vi "ADC SNR_new - Copy.vi"(8 "error in (no error)":errorcluster, 9 "Sequence parameters":string[][](array[string])=[["Min limit", "Max limit", "Register sheet file", "Register Sheet"], ["", "", "CC2600.xls", "TX_BLE;Trim"], ["Reg write (addr;value)", "Operating frequency [Hz]", "", ""], ["NA", "2.44G", "", ""]], 10 "Run type":i32, 11 "Method parameters":T4={"Dev"={"Do not disturb DUT"=FALSE, "XOSC"=32000000.0, "Board type"="", "EM"="", "Configure tempboard"=TRUE, "Device specific info"=[], "Generic Object"=refnum}, "Method"={"Run type"=1, "Test name"="Current LPM2 4", "Comment"="", "Results folder"="", "AFC"=enum."Off", "Method name"="Current LPM2 4", "Method results"={"Excel brief report"=FALSE, "Spotfire report"=FALSE, "Starfish report"=FALSE}, "Operator"="", "Reference time"=timestamp(0 s since 1904-01-01), "AFC delay"=0.0, "Initialization"=enum."Enabled", "MD5 Sum"="", "HW addon board"=enum."None", "AFC Regsheet"="", "AFC Regfile"=path "", "dummy"=0.0}, "Inst"={"Instr"={"PS1"={"Name"="", "GPIB address"="", "VISA session"=""}, "PS2"={"Name"="", "GPIB address"="", "VISA session"=""}, "TC1"={"Name"="", "GPIB address"="", "VISA session"=""}, "TC2"={"Name"="", "GPIB address"="", "VISA session"=""}, "SA1"={"Name"="", "GPIB address"="", "VISA session"=""}, "SA2"={"Name"="", "GPIB address"="", "VISA session"=""}, "SG1"={"Name"="", "GPIB address"="", "VISA session"=""}, "SG2"={"Name"="", "GPIB address"="", "VISA session"=""}, "SG3"={"Name"="", "GPIB address"="", "VISA session"=""}, "MI1"={"Name"="", "GPIB address"="", "VISA session"=""}, "MI2"={"Name"="", "GPIB address"="", "VISA session"=""}, "SW SA"={"Name"="", "Controller addr"=""}, "SW SG"={"Name"="", "Controller addr"=""}, "MI3"={"Name"="", "GPIB address"="", "VISA session"=""}}, "Switchbox"={"RF Path"=0, "Cal compensation"=enum."TX", "Switchbox gain mode"="", "State"=enum."TX"}, "Instr to control (i.e. SA1)"="Default", "Intrument info string"=""}, "Sequence parameters"=[["Weight", "Min Limit", "Max Limit", "Register Sheet", "", "", "", "", "", "", "", "", ""], ["Vital", "", "1", "LPM2", "", "", "", "", "", "", "", "", ""], ["Resolution", "Reg write (addr;value)", "Chip mode", "Range", "", "", "", "", "", "", "", "", ""], ["u", "NA", "", "auto", "", "", "", "", "", "", "", "", ""]], "Cond"={"Temp logged"=25.0, "VDD1_PS1_6V"=-999.0, "VDD2_PS1_25V"=-999.0, "VDD4_PS2_25V"=-999.0, "VDD3_PS2_6V"=-999.0}, "Meas config"={"X-axis inner loop index"=32000000, "Y-axis outer loop index"=32000000, "X-axis"=[], "Y-axis"=[], "X-axis array req size"=32000000, "Y-axis array req size"=32000000, "Param description"=[], "Use meas clust for reporting"=FALSE, "Parameter index (page)"=0, "X-axis name"="", "Y-axis name"=""}} {"Cond"."VDD3_PS2_6V" format="%.3f"; "Cond"."VDD4_PS2_25V" format="%.3f"; "Cond"."VDD2_PS1_25V" format="%.3f"; "Cond"."VDD1_PS1_6V" format="%.3f"; "Method"."dummy" format="%.1p"; "Method"."AFC delay" format="%.1p"; "Dev"."XOSC" format="%.3p"}) -> (0 "error out":errorcluster, 1 "End method error":T2, 2 "Short Results":string[](array[string])=["0.00", "0.00", "0.00", "0.00"], 3 "Result summary":string[][](array[string])=[["Critical", "Output Power@2405 MHz", "-3", "4", "dBm"], ["Critical", "Output Power@2410 MHz", "-3", "4", "dBm"]])   [LabVIEW 2019]
doc: "[AutoDocStart]Performs crystal accuracy measurements. Measures the offset from ideal frequency. Primarily used for tuning XOSC capacitors and verifying XOSC trims.\n\nSweeping parameters: operating frequency, OSC override value and VDDR level\n\nResults: Offset frequency in ppm[AutoDocEnd]"
uses:
  User Lib/Utilities/Cluster definitions/Method input.ctl
  User Lib/Utilities/Cluster definitions/Device specific info.ctl
  User Lib/Utilities/Controls/Automatic Frequency Compensation types.ctl
  User Lib/Utilities/Controls/Method Reports.ctl
  User Lib/Utilities/Cluster definitions/Method Initialization.ctl
  User Lib/Utilities/Controls/HW addon boards.ctl
  User Lib/Utilities/Cluster definitions/Instr clust.ctl
  User Lib/Utilities/Switchbox control/SwitchBox_State._ENUMctl.ctl
  User Lib/Utilities/Cluster definitions/End method error cluster.ctl
  User Lib/Utilities/Cluster definitions/DUT vdd control.ctl
  User Lib/Utilities/Cluster definitions/DUT VDD4.ctl
  User Lib/Utilities/Cluster definitions/DUT VDD3.ctl
  User Lib/Utilities/Cluster definitions/DUT VDD2.ctl
  User Lib/Utilities/Cluster definitions/DUT VDD1.ctl
  User Lib/Generic chip methods/Classes/Generic_EM/Chameleon/Loki/Loki.lvclass
  <vilib>/Utility/error.llb/Clear Errors.vi
  User Lib/Generic chip methods/Classes/Generic_EM/Chameleon/65nm.lvclass
  C:/Kharon/User Lib/Generic chip methods/Classes/Generic_EM/Generic_EM/Generic_EM.lvclass
  User Lib/Generic chip methods/board_to_chip_type.vi
  User Lib/Generic chip methods/Classes/Get_Class_init.vi
  User Lib/Generic chip methods/Classes/Generic_EM/Generic_EM/Generic_EM.lvclass
panel:
  in  "Tab Control":T1(tab)
  out "Dynamic Parameters":T3={"SNR"=nan, "SNRD"=nan, "THD"=nan, "ENOB (SNRD)"=nan, "SFDR"=nan, "ENOB (SNR)"=nan, "Noise Power"=nan, "Signal power"=nan} {"Signal power" format="%.6f"; "Noise Power" format="%.2f"; "ENOB (SNR)" format="%.2f"; "SFDR" format="%.2f"; "ENOB (SNRD)" format="%.2f"; "THD" format="%.2f"; "SNRD" format="%.2f"; "SNR" format="%.2f"}
  out "ADC samples":u32[](array[numeric])
  out "Output Response [All DUTs]":u32[][](array[numeric])
  out "SNR":dbl
  out "Noise Power":dbl
  out "Signal power":dbl
  out "ENOB (SNR)":dbl
  out "detected Throughput":dbl=200065.4236150998
  # "°C"
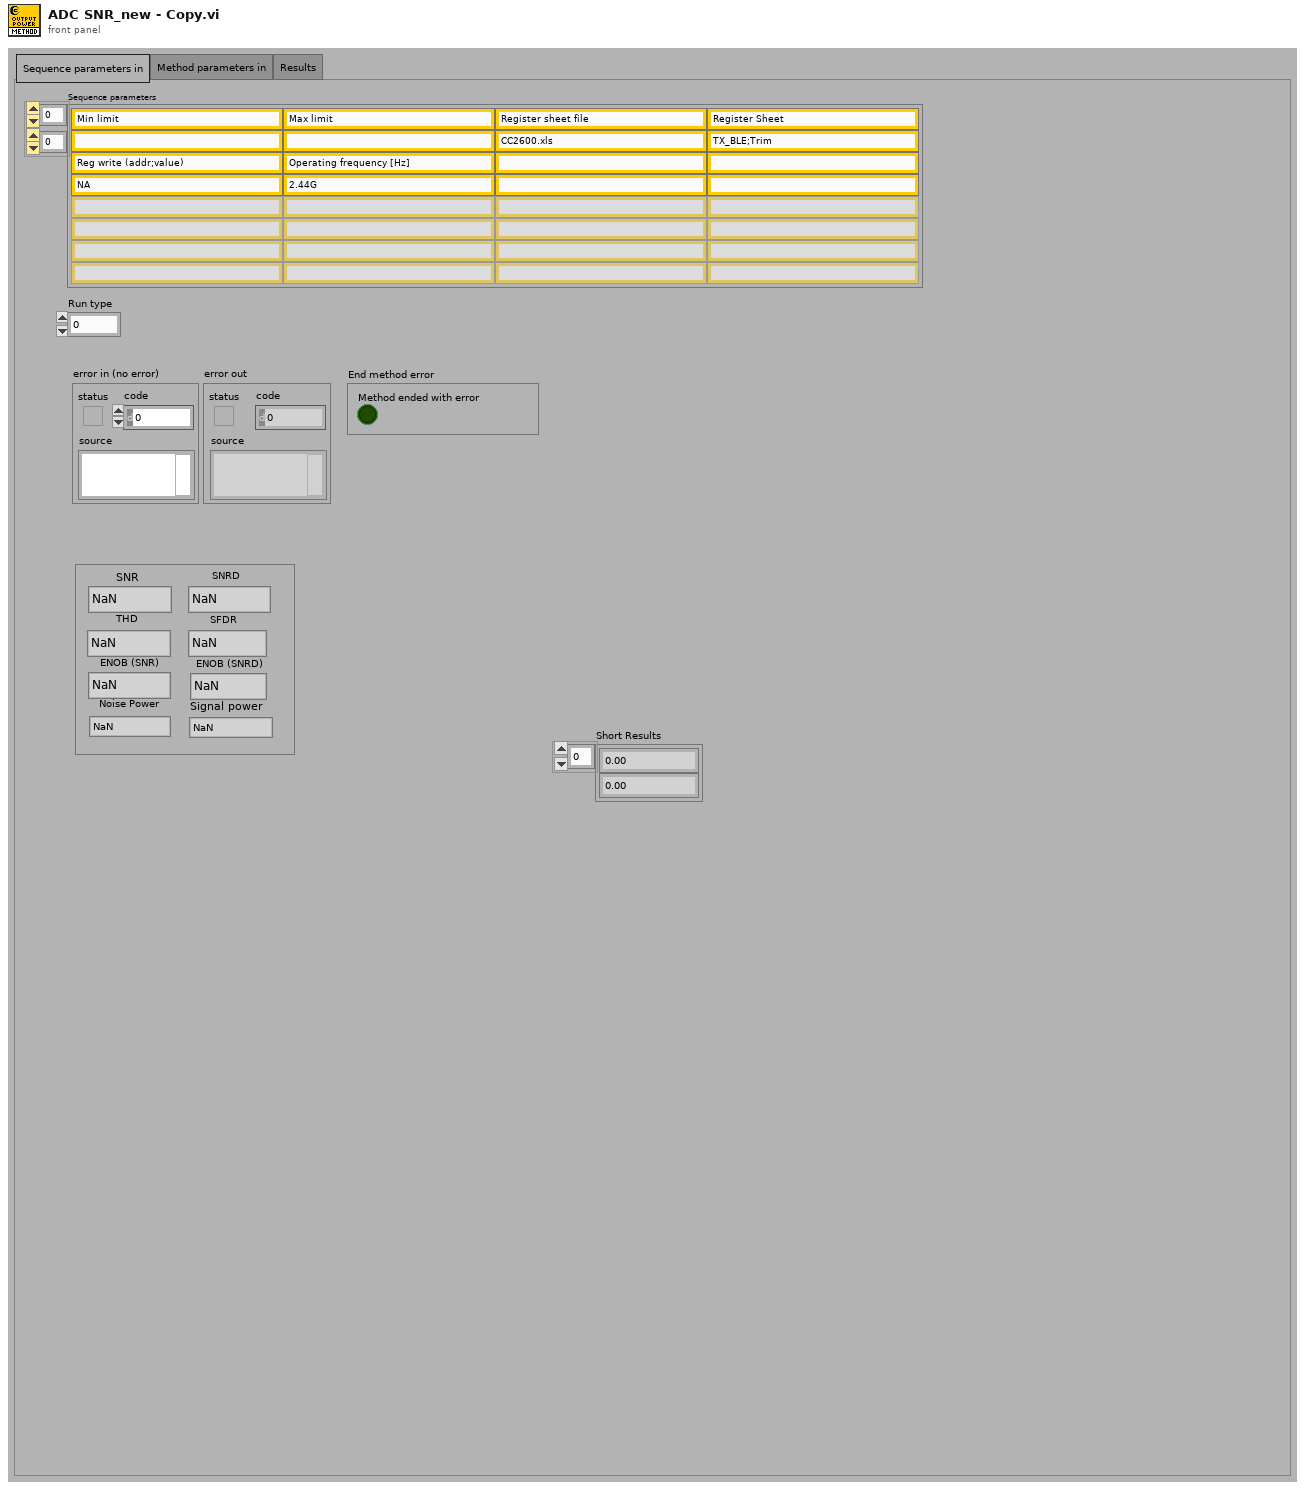
[diagram p1: front panel]
types:
  T1 = enum32{"Sequence parameters in", "Method parameters in", "Results"}
  T2 = typedef "End method error cluster.ctl" = cluster{"Method ended with error":bool}
  T3 = cluster{"SNR":dbl, "SNRD":dbl, "THD":dbl, "ENOB (SNRD)":dbl, "SFDR":dbl, "ENOB (SNR)":dbl, "Noise Power":dbl, "Signal power":dbl}
  T4 = typedef "Method input.ctl" = cluster{"Dev":cluster{"Do not disturb DUT":bool, "XOSC":dbl, "Board type":string, "EM":string, "Configure tempboard":bool, "Device specific info":T5[], "Generic Object":refnum<class>}, "Method":cluster{"Run type":i32, "Test name":string, "Comment":string, "Results folder":string, "AFC":T6, "Method name":string, "Method results":T7, "Operator":string, "Reference time":timestamp, "AFC delay":dbl, "Initialization":T8, "MD5 Sum":string, "HW addon board":T9, "AFC Regsheet":string, "AFC Regfile":path, "dummy":dbl}, "Inst":T10, "Sequence parameters":string[][], "Cond":cluster{"Temp logged":dbl, "VDD1_PS1_6V":dbl, "VDD2_PS1_25V":dbl, "VDD4_PS2_25V":dbl, "VDD3_PS2_6V":dbl}, "Meas config":cluster{"X-axis inner loop index":i32, "Y-axis outer loop index":i32, "X-axis":string[], "Y-axis":string[], "X-axis array req size":i32, "Y-axis array req size":i32, "Param description":string[][], "Use meas clust for reporting":bool, "Parameter index (page)":i32, "X-axis name":string, "Y-axis name":string}}
  T5 = typedef "Device specific info.ctl" = cluster{"EM number":u8, "IP address":string, "Enabled":bool, "Slot no":u8, "RF path":u8, "EM name":string, "Wafer info":string, "AFC frequency ppm":dbl, "Register writes":string[][], "Meas data":string[][][], "Device comment":string}
  T6 = typedef "Automatic Frequency Compensation types.ctl" = enum16{"Off", "Compensate Instrument frequency", "Compensate DUT frequency", "Predictive - Compensate Instrument frequency", "Predictive - Compensate DUT frequency", "Do not skip re-init - Compensate Instrument frequency", "Do not skip re-init - Compensate DUT frequency"}
  T7 = typedef "Method Reports.ctl" = cluster{"Excel brief report":bool, "Spotfire report":bool, "Starfish report":bool}
  T8 = typedef "Method Initialization.ctl" = enum16{"Enabled", "Skip Instr and Device Init", "Enabled with Separate Flash", "Set PS, Device Init and Skip Instr Init", "Skip Device Init"}
  T9 = typedef "HW addon boards.ctl" = enum16{"None", "Current meas 5EM", "Stresstest 10EM"}
  T10 = typedef "Instr clust.ctl" = cluster{"Instr":cluster{"PS1":cluster{"Name":string, "GPIB address":string, "VISA session":refnum<visa-resource-name>}, "PS2":cluster{"Name":string, "GPIB address":string, "VISA session":refnum<visa-resource-name>}, "TC1":cluster{"Name":string, "GPIB address":string, "VISA session":refnum<visa-resource-name>}, "TC2":cluster{"Name":string, "GPIB address":string, "VISA session":refnum<visa-resource-name>}, "SA1":cluster{"Name":string, "GPIB address":string, "VISA session":refnum<visa-resource-name>}, "SA2":cluster{"Name":string, "GPIB address":string, "VISA session":refnum<visa-resource-name>}, "SG1":cluster{"Name":string, "GPIB address":string, "VISA session":refnum<visa-resource-name>}, "SG2":cluster{"Name":string, "GPIB address":string, "VISA session":refnum<visa-resource-name>}, "SG3":cluster{"Name":string, "GPIB address":string, "VISA session":refnum<visa-resource-name>}, "MI1":cluster{"Name":string, "GPIB address":string, "VISA session":refnum<visa-resource-name>}, "MI2":cluster{"Name":string, "GPIB address":string, "VISA session":refnum<visa-resource-name>}, "SW SA":cluster{"Name":string, "Controller addr":string}, "SW SG":cluster{"Name":string, "Controller addr":string}, "MI3":cluster{"Name":string, "GPIB address":string, "VISA session":refnum<visa-resource-name>}}, "Switchbox":cluster{"RF Path":i32, "Cal compensation":enum16{"TX", "RX", "Interferer", "No compensation", "Interferer2"}, "Switchbox gain mode":string, "State":T11}, "Instr to control (i.e. SA1)":string, "Intrument info string":string}
  T11 = typedef "SwitchBox_State._ENUMctl.ctl" = enum16{"TX", "RX", "SP:TX", "SP:RX", "SW:TX", "SW:RX"}
  T12 = cluster{"Fundamental Frequency":dbl, "Sampling Frequncy":dbl, "No of Harmonics":u8, "Window":enum16{"None ", "Hanning", "Hamming", "Blackman-Harris", "Exact Blackman", "Blackman", "Flat Top", "4 Term B-Harris ", "7 Term B-Harris"}, "Blackman (fundamental power) bins)":dbl}
  T13 = cluster{"Save INL/DNL Plot(Ramp)":bool, "Save SNR Plot":bool, "Save INL/DNL Plot(Sine)":bool, "Save INL/DNL Raw Data(Ramp)":bool, "Save SNR Raw Data":bool, "Save INL/DNL Raw Data(Sine)":bool, "Save DC Raw data":bool, "Save  Raw Data(Sine)":bool}
  T14 = typedef "DUT vdd control.ctl" = cluster{"VDD4 config":T15, "VDD3 config":T16, "VDD2 config":T17, "VDD1 config":T18}
  T15 = typedef "DUT VDD4.ctl" = u16
  T16 = typedef "DUT VDD3.ctl" = u16
  T17 = typedef "DUT VDD2.ctl" = u16
  T18 = typedef "DUT VDD1.ctl" = u16
  T19 = cluster{"Path to Save plot":path, "Path to Raw Data plot":path}
  T20 = enum32{"NI Card Settings", "Memory Read Setting", "DC Capture", "ADC Ramp", "ADC Sine", "SNR", "Cap Calibration"}
  T21 = enum32{"Read from Memory", "Read .dat file", "NI Card Capture", "None"}
  T22 = typedef "TFW ResponseData.ctl" = cluster{"errorCode":u32, "executionTime":u32, "processedCmdWord":u32, "responsePar":u32[], "actionCode":u32, "cmdStatus":u16}
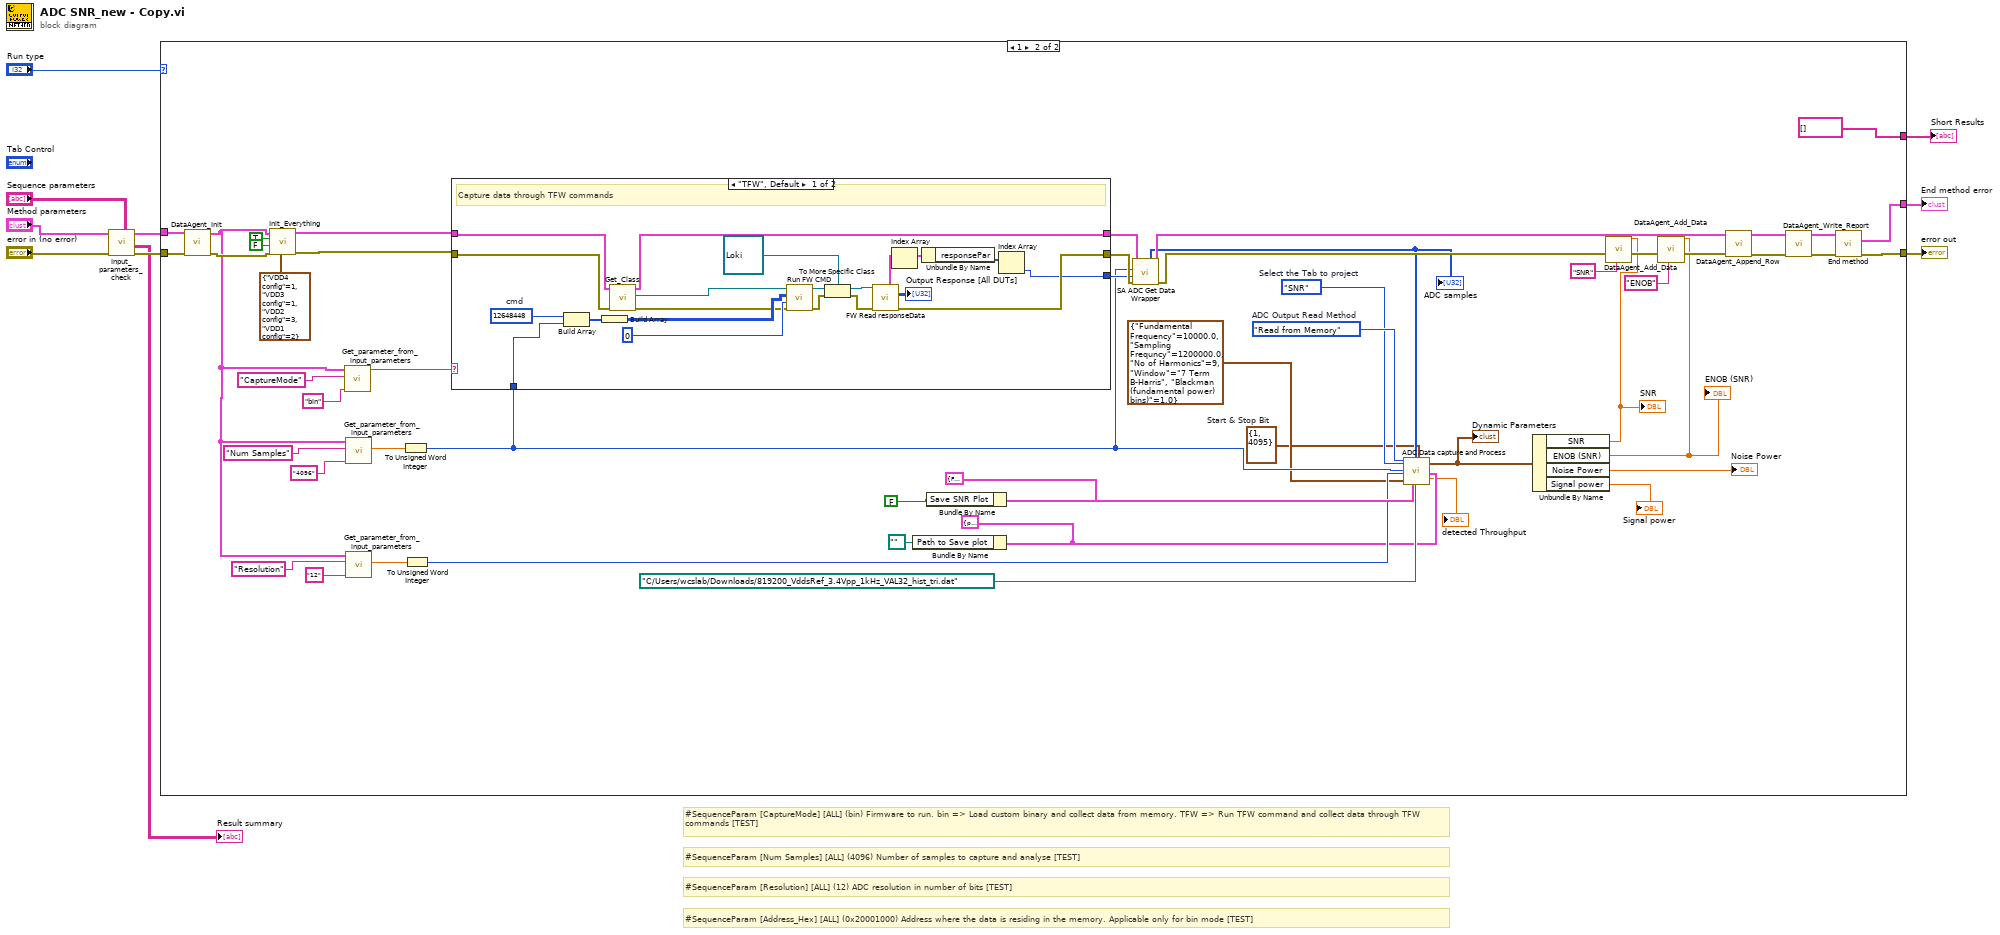
[diagram p0: block diagram]
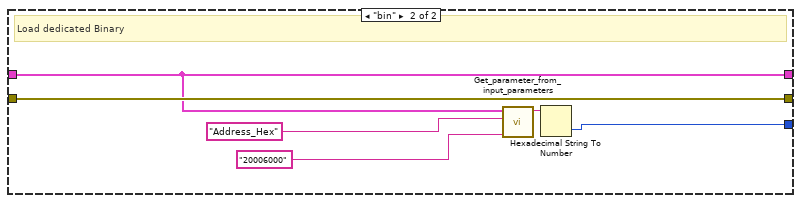
[diagram p3: hidden frame]
diagram:
  # "#SequenceParam [Num Samples] [ALL] (4096) Number of samples to capture and analyse [TEST]"
  # "#SequenceParam [CaptureMode] [ALL] (bin) Firmware to run. bin => Load custom binary and collect data from memory. TFW => Run TFW command and collect data through TFW commands [TEST]"
  # "#SequenceParam [Address_Hex] [ALL] (0x20001000) Address where the data is residing in the memory. Applicable only for bin mode [TEST]"
  # "#SequenceParam [Resolution] [ALL] (12) ADC resolution in number of bits [TEST]"
  n1 = call "Input_parameters_check.vi"("Sequence parameters"="Sequence parameters", "error in"="error in (no error)", "Method cluster in"="Method parameters") -> ("error out"=w9:errorcluster, "Result summary"=→"Result summary":string[][], "Method cluster out"=w5:T4)  [unwired: 6 in]
  n2 = case shown="1" "Run type" {
    tunnel: w9 -> [w11 w60]
    tunnel: [w11 w64] -> w10
    tunnel: w5 -> [_ w61]
    tunnel: [_ w63] -> w4
    tunnel: [_ string[] []] -> w1
    frame 0, Default {
      # "Run type 0 is only for formatting the result summary"
    }
    frame 1 {
      w13 = cluster{"Start":i32, "Stop":i32} {"Start"=1, "Stop"=4095}  # Start & Stop Bit
      w14 = T19 {"Path to Save plot"=path "D:/Tenor_176P/DYN_PAR_C004/DAT/D001_TEMPP30C_VDD1.2_VDDA3.3_16B_SE_ADCA__vicA_aggX_PLT_CAP_200821_1740_33.jpg", "Path to Raw Data plot"=path "D:/Tenor_176P/DYN_PAR_C004/DAT/D001_TEMPP30C_VDD1.2_VDDA3.3_16B_SE_ADCA__vicA_aggX_RAW_DAT_200821_1740_33.csv"} ("path to save")
      w50 = T20."SNR"  # Select the Tab to project
      w51 = T21."Read from Memory"  # ADC Output Read Method
      n3 = call "DataAgent_Init.vi"("error in (no error)"=w60, "Method cluster in"=w61) -> ("error out"=w59:errorcluster, "Method cluster out"=w30:T4)  [unwired: 8 in]
      n4 = call "Init_Everything.vi"("VDD config"=T14 {"VDD4 config"=1, "VDD3 config"=1, "VDD2 config"=3, "VDD1 config"=2}, "error in"=w59, "Support current measurement?"=FALSE, "Override VDD Config"=TRUE, "Method cluster In"=w30) -> ("error out"=w56:errorcluster, "Method cluster out"=w55:T4)  [unwired: 3 in, 2 out]
      n5 = call "Get_parameter_from_input_parameters.vi"("Default value (used if not specified on Front Panel)"="bin", "Parameter name"="CaptureMode" ("SA_ param name"), "Method cluster (if input param empty)"=w30) -> ("value as String"=w42:string)  [unwired: 2 in, 6 out]
      n6 = call "Get_parameter_from_input_parameters.vi"("Default value (used if not specified on Front Panel)"="4096", "Parameter name"="Num Samples" ("SA_ param name"), "Method cluster (if input param empty)"=w30) -> ("value as DBL"=w33:dbl)  [unwired: 2 in, 6 out]
      n7 = call "Get_parameter_from_input_parameters.vi"("Default value (used if not specified on Front Panel)"="12", "Parameter name"="Resolution" ("SA_ param name"), "Method cluster (if input param empty)"=w30) -> ("value as DBL"=w52:dbl)  [unwired: 2 in, 6 out]
      n8 = To Unsigned Word Integer(number=w33) -> (unsigned 16bit integer=w29:u16)
      n9 = To Unsigned Word Integer(number=w52) -> (unsigned 16bit integer=w45:u16)
      n10 = case shown="\"TFW\", Default" w42 {
        tunnel: [w85 w86] -> w36
        tunnel: [w78 w91] -> w35
        tunnel: w56 -> [w77 w91]
        tunnel: w55 -> [w84 w86]
        tunnel: [w65 w87] -> w34
        tunnel: w29 -> [w81 _]
        frame "TFW", Default {
          w82 = u32 12648448  # cmd
          # "Capture data through TFW commands"
          n11 = Build Array(w82, w81) -> (w80:u32[])
          n12 = Build Array(w80) -> (w79:u32[][])
          n13 = call "Get_Class.vi"("error in (no error)"=w77, "Method cluster in"=w84) -> ("error out"=w75:errorcluster, "Class Out"=w74:refnum<class "Generic_EM.lvclass">, "Method cluster out"=w85:T4)  [unwired: 6 in, 1 out]
          n14 = call-dynamic "Run FW CMD.vi"("error in (no error)"=w75, "Handler"=u8 0, "cmdBuf"=w79, "Generic_EM in"=w74) -> ("error out"=w70:errorcluster, "Generic_EM out"=w73:refnum<class "Generic_EM.lvclass">)  [unwired: 6 in]
          n15 = To More Specific Class(target class=refnum<class "Loki.lvclass"> refnum ("Loki in"), reference=w73, error in=w70) -> (specific class reference=w71:refnum<class "Loki.lvclass">, error out=w69:errorcluster)
          n16 = call "FW Read responseData.vi"("error in (no error)"=w69, "Loki in"=w71) -> ("error out"=w78:errorcluster, "Output Response [All DUTs]"=→"Output Response [All DUTs]":u32[][], "Response"=w67:T22[])  [unwired: 6 in, 1 out]
          n17 = Index Array(array=w67) -> (element=w68:T22)  [unwired: 1 in]
          n18 = Unbundle By Name(w68) -> ("responsePar"=w66:u32[])
          n19 = Index Array(array=w66) -> (element=w65:u32)  [unwired: 1 in]
        }
        frame "bin" {
          # "Load dedicated Binary"
          n20 = call "Get_parameter_from_input_parameters.vi"("Default value (used if not specified on Front Panel)"="20006000", "Parameter name"="Address_Hex" ("SA_ param name"), "Method cluster (if input param empty)"=w86) -> ("value as String"=w90:string)  [unwired: 2 in, 6 out]
          n21 = Hexadecimal String To Number(string=w90) -> (number=w87:u32)  [unwired: 2 in, 1 out]
        }
      }
      n22 = Bundle By Name(cluster=w14, "Path to Save plot"=path "") -> ()  [unwired: 1 out]
      n23 = Bundle By Name(cluster=T13 {"Save INL/DNL Plot(Ramp)"=FALSE, "Save SNR Plot"=FALSE, "Save INL/DNL Plot(Sine)"=FALSE, "Save INL/DNL Raw Data(Ramp)"=FALSE, "Save SNR Raw Data"=FALSE, "Save INL/DNL Raw Data(Sine)"=FALSE, "Save DC Raw data"=FALSE, "Save  Raw Data(Sine)"=FALSE} ("Save data"), "Save SNR Plot"=FALSE) -> (w48:T13)
      n24 = call "SA ADC Get Data Wrapper.vi"("error in"=w35, "Data Address"=w34, "Num Samples"=w29, "Method cluster in"=w36) -> ("error out"=w39:errorcluster, "output cluster"=w38:T4, "ADC samples"=w37:u32[])  [unwired: 2 in, 3 out]
      "ADC samples" <- w37
      n25 = call "ADC Data capture and Process.vi"("ADC Output Read Method"=w51, "Select the Tab to project"=w50, "No.of samples(SNR)"=w29, "Resolution"=w45, "Inputs for Dyanmic para"=T12 {"Fundamental Frequency"=10000.0, "Sampling Frequncy"=1200000.0, "No of Harmonics"=9, "Window"=enum."7 Term B-Harris", "Blackman (fundamental power) bins)"=1.0}, "Save data"=w48, "Waveform"=w37, "Path to Read"=path "C:/Users/wcslab/Downloads/819200_VddsRef_3.4Vpp_1kHz_VAL32_hist_tri.dat", "Start & Stop Bit"=w13, "path to save"=w14) -> ("detected Throughput"=→"detected Throughput":dbl, "Dynamic Parameters"=w19:T3)  [unwired: 11 in, 5 out]
      "Dynamic Parameters" <- w19
      n26 = Unbundle By Name(w19) -> ("SNR"=w18:dbl, "ENOB (SNR)"=w17:dbl, "Noise Power"=→"Noise Power":dbl, "Signal power"=→"Signal power":dbl)
      "SNR" <- w18
      "ENOB (SNR)" <- w17
      n27 = call "DataAgent_Add_Data.vi"("ColumnName"="SNR" ("Default Value"), "Data"=w18, "error in (no error)"=w39) -> ("error out"=w25:errorcluster)  [unwired: 8 in]
      n28 = call "DataAgent_Add_Data.vi"("ColumnName"="ENOB" ("Default Value"), "Data"=w17, "error in (no error)"=w25) -> ("error out"=w24:errorcluster)  [unwired: 8 in]
      n29 = call "DataAgent_Append_Row.vi"("error in (no error)"=w24, "Method cluster in"=w38) -> ("error out"=w27:errorcluster, "Method cluster out"=w28:T4)  [unwired: 8 in]
      n30 = call "DataAgent_Write_Report.vi"("error in (no error)"=w27, "Method cluster in"=w28) -> ("error out"=w58:errorcluster, "Method cluster out"=w57:T4)  [unwired: 8 in]
      n31 = call "End method.vi"("error in"=w58, "Method cluster in"=w57) -> ("error out"=w64:errorcluster, "End method error"=w63:T2)  [unwired: 7 in, 1 out]
    }
  }
  "error out" <- w10
  "End method error" <- w4
  "Short Results" <- w1
